vi "NativeSubTemplate_Init.vi"(0 "object in":refnum<class "NativeSubTemplate.lvclass">, 5 "Error In":errorcluster) -> (14 "object out":refnum<class "NativeSubTemplate.lvclass">, 19 "Error Out":errorcluster)   [LabVIEW 2020, in "NativeSubTemplate.lvclass"]
uses:
  <resource>/Framework/Providers/Open_GDS/ClassProviders/Provider_LvNativeClass/Templates/NativeSubTemplate/NativeSubTemplate.lvclass
  C:/Program Files (x86)/National Instruments/LabVIEW 2020/resource/Framework/Providers/Open_GDS/ClassProviders/Provider_LvNativeClass/Templates/NativeBaseTemplate/NativeBaseTemplate.lvclass
  <resource>/Framework/Providers/Open_GDS/ClassProviders/Provider_LvNativeClass/Templates/NativeSubTemplate/NativeSubTemplate.lvclass/NativeSubTemplate.ctl
  <resource>/Framework/Providers/Open_GDS/ClassProviders/Provider_LvNativeClass/Templates/NativeBaseTemplate/NativeBaseTemplate.lvclass
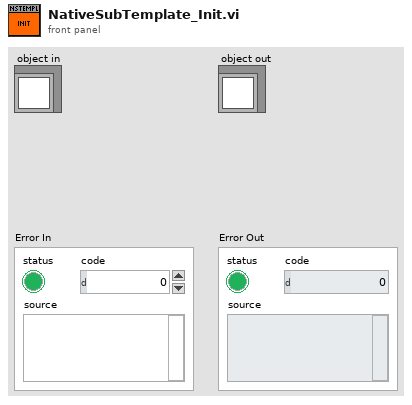
[diagram p1: front panel]
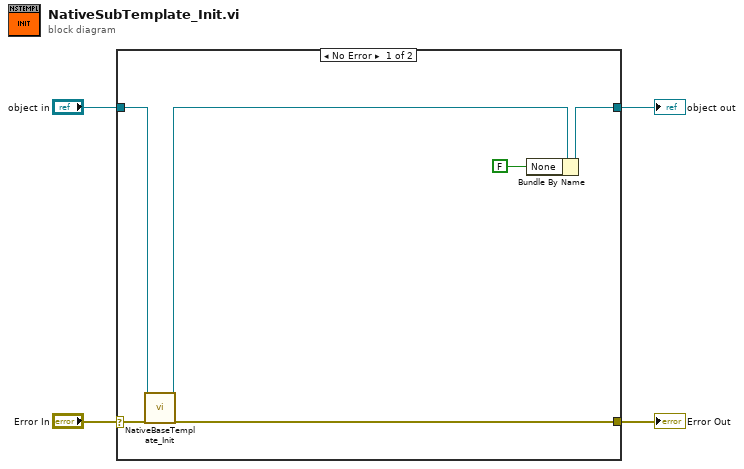
[diagram p0: block diagram]
diagram:
  n1 = case shown="No Error" "Error In" {
    selector: "Error In" -> [w8 w11]
    tunnel: [w10 w12] -> w4
    tunnel: "object in" -> [w6 w12]
    tunnel: [w7 w11] -> w1
    frame No Error {
      n2 = call <resource>:"NativeBaseTemplate_Init.vi"("object in"=w6, "Error In"=w8) -> ("object out"=w5:refnum<class "NativeSubTemplate.lvclass">, "Error Out"=w7:errorcluster)  [unwired: 16 in]
      n3 = Bundle By Name(cluster=w5, "None"=FALSE) -> (w10:refnum<class "NativeSubTemplate.lvclass">)
    }
    frame Error {
    }
  }
  "object out" <- w4
  "Error Out" <- w1
